vi "Operation.vi"(8 "Error In":errorcluster, 11 "Multiply in":refnum<class "Multiply.lvclass">) -> (0 "Error out":errorcluster, 2 "C":dbl, 3 "Multiply out":refnum<class "Multiply.lvclass">)   [LabVIEW 2019, in "Multiply.lvclass"]
uses:
  Multiply.lvclass
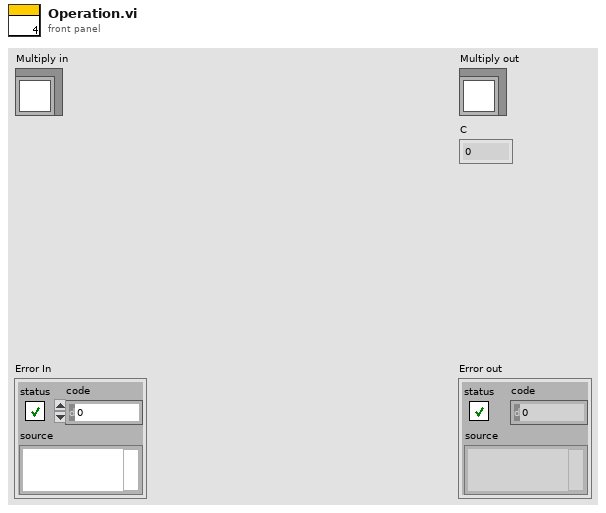
[diagram p1: front panel]
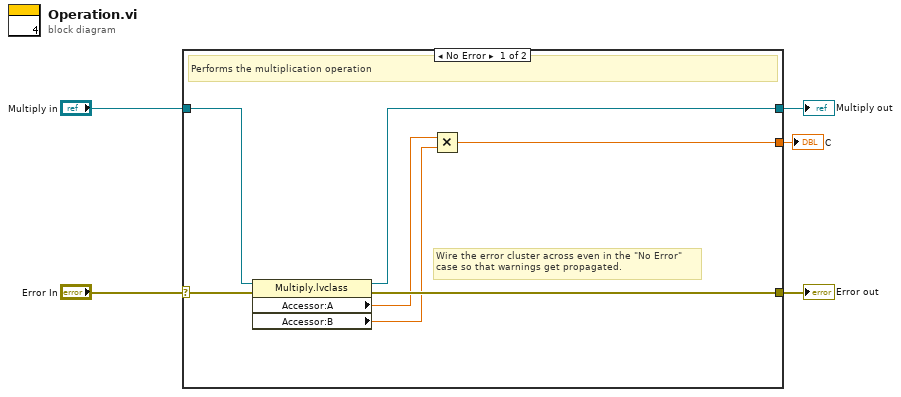
[diagram p0: block diagram]
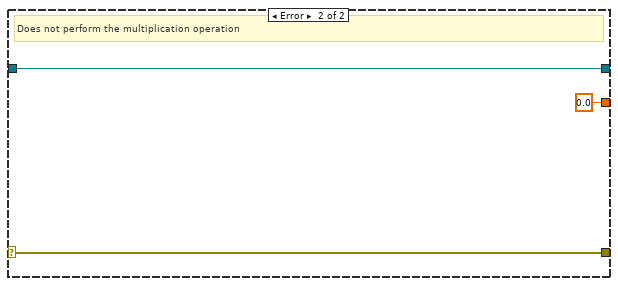
[diagram p2: hidden frame]
diagram:
  n1 = case shown="No Error" "Error In" {
    selector: "Error In" -> [w12 w15]
    tunnel: [w10 w15] -> w4
    tunnel: [w6 w14] -> w2
    tunnel: "Multiply in" -> [w9 w14]
    tunnel: [w11 0.0] -> w1
    frame No Error {
      # "Wire the error cluster across even in the \"No Error\"\ncase so that warnings get propagated."
      # "Performs the multiplication operation"
      n2 = property class="Multiply.lvclass"(reference=w9, error in=w12) -> (reference out=w6:refnum<class "Multiply.lvclass">, error out=w10:errorcluster, "Accessor:A"=w8:dbl, "Accessor:B"=w7:dbl)
      n3 = Multiply(x=w8, y=w7) -> (x*y=w11:dbl)
    }
    frame Error {
      # "Does not perform the multiplication operation"
    }
  }
  "Error out" <- w4
  "Multiply out" <- w2
  "C" <- w1
